vi "PH_ImageOperator.write PSDB Position data.vi"(0 "i ref in":refnum<vi>, 5 "error in":errorcluster) -> (14 "i ref out":refnum<vi>, 16 "Position Boolean data":T1[](array[typedef]), 17 "Position Numeric data":T3[](array[typedef]), 18 "Position String data":T2[](array[typedef]), 19 "error out":errorcluster)   [LabVIEW 2014, in "PH_ImageOperator.lvlib"]
uses:
  PH_ImageOperator.lvlib
  PH_PSDBWriter/PH_PSDBWriter.Numeric dataset.ctl
  PH_PSDBWriter/PH_PSDBWriter.String dataset.ctl
  PH_PSDBWriter/PH_PSDBWriter.Boolean dataset.ctl
  PH_StatusHandler/PH_StatusHandler.Status.ctl
  PH_PSDBWriter/PH_PSDBWriter.lvlib
  PH_StatusHandler/PH_StatusHandler.lvlib
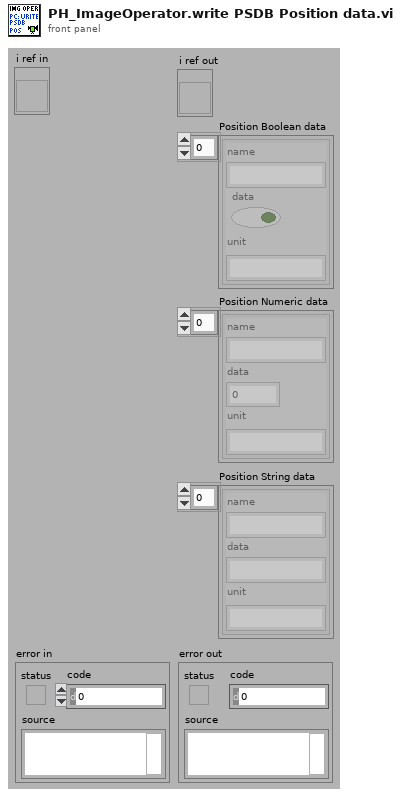
[diagram p1: front panel]
types:
  T1 = typedef "PH_PSDBWriter.lvlib/PH_PSDBWriter.Boolean dataset.ctl" = cluster{"name":string, "data":bool, "unit":string}
  T2 = typedef "PH_PSDBWriter.lvlib/PH_PSDBWriter.String dataset.ctl" = cluster{"name":string, "data":string, "unit":string}
  T3 = typedef "PH_PSDBWriter.lvlib/PH_PSDBWriter.Numeric dataset.ctl" = cluster{"name":string, "data":dbl, "unit":string}
  T4 = typedef "PH_ImageOperator.lvlib/PH_ImageOperator.i attribute.ctl" = cluster{"GUI Refs":cluster{"Delete":refnum<vi>, "Calibration status":refnum<vi>, "BI subtracted":refnum<vi>, "calc Energy":refnum<vi>, "Energy: expected value":refnum<vi>, "Energy: Tolerance":refnum<vi>, "Energy calculated":refnum<vi>, "Energy":refnum<vi>, "calc Beam Anal":refnum<vi>, "Maj Diam 1/esquare":refnum<vi>, "Min Diam 1/esquare":refnum<vi>, "Azi Angle":refnum<vi>, "Min/Maj Diam esquare":refnum<vi>, "Beam analysed":refnum<vi>, "CoG - x":refnum<vi>, "CoG - y":refnum<vi>, "BA: Method":refnum<vi>, "BA: Steps":refnum<vi>, "BA: Factor":refnum<vi>, "calc Traces":refnum<vi>, "Traces: Fit Gauss":refnum<vi>, "Traces calculated":refnum<vi>, "Maj FWHM":refnum<vi>, "Min FWHM":refnum<vi>, "Major Trace":refnum<vi>, "Minor Trace":refnum<vi>, "Maj Fit Order":refnum<vi>, "Min Fit Order":refnum<vi>, "Position calculated":refnum<vi>, "Position":refnum<vi>, "Type":refnum<vi>, "Center":refnum<vi>, "exp - X":refnum<vi>, "exp - Y":refnum<vi>, "Tolerance":refnum<vi>, "f":refnum<vi>, "M":refnum<vi>, "D":refnum<vi>, "q":refnum<vi>, "Dummy Method":refnum<vi>, "Dummy Type":refnum<vi>, "Global On":refnum<vi>, "Traces: No offset":refnum<vi>, "Maj 99%":refnum<vi>, "Min 99%":refnum<vi>, "GUI FF Image":refnum<vi>, "calc Fill Factor":refnum<vi>, "FF calculated":refnum<vi>, "Fill Factor: Filter?":refnum<vi>, "FF: Damage Threshold":refnum<vi>, "FF: Threshold":refnum<vi>, "FF: max allow. Energy":refnum<vi>, "FF: Fillfactor":refnum<vi>, "Calibration data":refnum<vi>}, "List of GUIs":string[], "Calibration":cluster{"Status":T5, "Calibration data":T6, "Calibration Data File":path}, "Final Image":cluster{"BI Subtraction Failure":bool}, "Energy":cluster{"on":bool, "expected value [mJ]":dbl, "Tolerance [%]":dbl, "State":T5, "Energy [mJ]":dbl, "Unit":string, "calculated @":timestamp}, "Beam Analysis":cluster{"on":bool, "Data":T7, "Method":bool, "Steps":i32, "Factor":i32, "ROI":cluster{"Left":i32, "Top":i32, "Right":i32, "Bottom":i32}, "analysed @":timestamp}, "Trace Analysis":cluster{"on":bool, "Fit on":bool, "Maj FWHM":dbl, "Min FWHM":dbl, "Maj Fit Order":i32, "Min Fit Order":i32, "No Offset":bool, "Maj 99%":dbl, "Min 99%":dbl, "Traces":cluster{"XScaleName":string, "Y Scale Minimum":sgl, "Y Scale Maximum":sgl, "X Scale Minimum":sgl, "X Scale Maximum":sgl, "Traces":cluster{"Index":sgl[], "Trace":dbl[]}[]}[], "analysed @":timestamp}, "Position Analysis":cluster{"on":bool, "exp - X":i32, "exp - Y":i32, "focal length [mm]":dbl, "Magnification":dbl, "Delta":dbl, "Theta":dbl, "Tolerance":dbl, "Type":bool, "analysed @":timestamp}, "Fill Factor":cluster{"on":bool, "Filter on?":bool, "Threshold":dbl, "Damage Threshold [J/cm²]":dbl, "Fillfactor":dbl, "Max. allowed Energy [J]":dbl, "calculated @":timestamp}, "Statistician Service ID":i32, "Images":cluster{"Background":T8, "OP":T8, "GUI":T8, "BA: ROI":T8, "Trace: Turn":T8, "FF: Main":T8, "FF: Help":T8, "PSDB: BG":T8, "PSDB: OP":T8, "PSDB: FF":T8}}
  T5 = typedef "PH_StatusHandler.lvlib/PH_StatusHandler.Status.ctl" = i16
  T6 = typedef "PH_ImageCalibrator.lvlib/PH_ImageCalibrator.Calibration Data.ctl" = cluster{"Date":string, "Time":string, "Cam Settings":cluster{"Cam ID":string, "Gain":dbl, "Brightness":dbl, "Shutter":dbl, "Cam Error":bool, "Mode":i32}, "Background Image":cluster{"Image":dbl[][], "Image Error":bool}, "Linear Calibration":cluster{"Calibration Factor":dbl, "not mm or mrad":bool}, "Energy Calibration":cluster{"Calibration Factor":dbl, "no mJ":bool}}
  T7 = typedef "PH_ImageOperator.lvlib/PH_ImageOperator.Beam Analysis Data.ctl" = cluster{"CoG-x":sgl, "CoG-y":sgl, "Maj Dim":dbl, "Min Dim":dbl, "Ellipticity":dbl, "Azimuth Angle [rad]":dbl, "Azi Angle rel to Maj?":bool}
  T8 = typedef "IMAQ Image.ctl" = refnum<image>
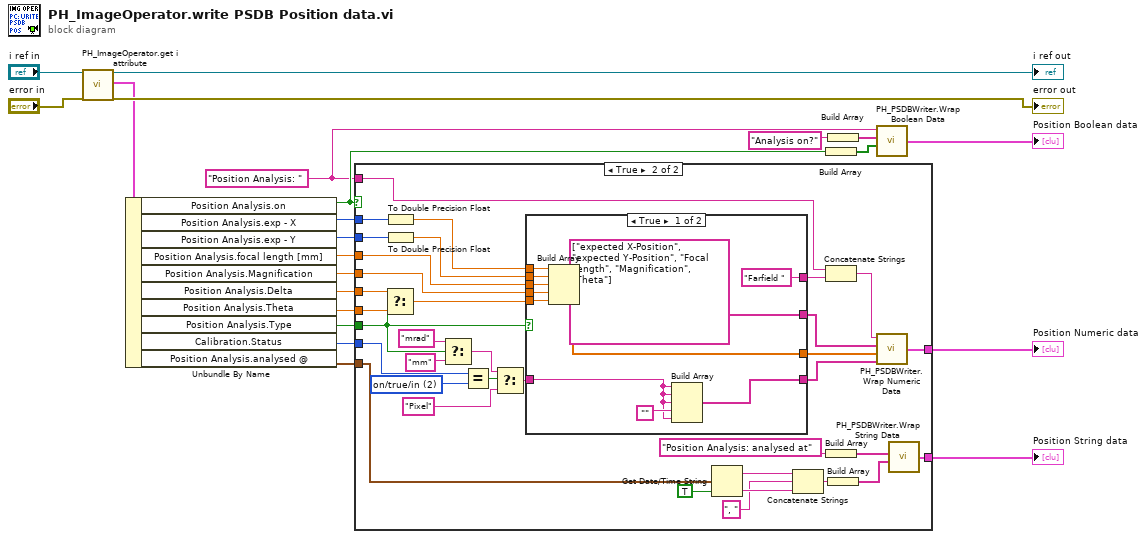
[diagram p0: block diagram]
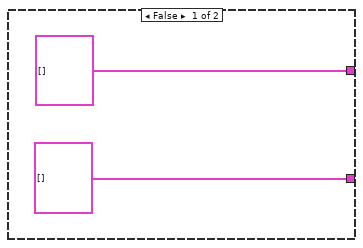
[diagram p2: hidden frame]
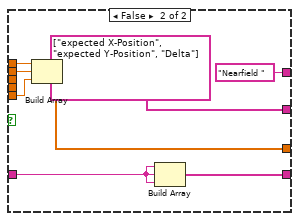
[diagram p3: hidden frame]
diagram:
  w3 = "Position Analysis: " ("string")
  n1 = call "PH_ImageOperator.get i attribute.vi"("i ref in"="i ref in", "error in (no error)"="error in") -> ("i ref out"=→"i ref out":refnum<vi>, "i attribute"=w17:T4, "error out"=→"error out":errorcluster)  [unwired: 15 in]
  n2 = Unbundle By Name(w17) -> ("Position Analysis.on"=w6:bool, "Position Analysis.exp - X"=w16:i32, "Position Analysis.exp - Y"=w15:i32, "Position Analysis.focal length [mm]"=w14:dbl, "Position Analysis.Magnification"=w13:dbl, "Position Analysis.Delta"=w12:dbl, "Position Analysis.Theta"=w11:dbl, "Position Analysis.Type"=w10:bool, "Calibration.Status"=w9:T5, "Position Analysis.analysed @"=w8:timestamp)
  n3 = case shown="True" w6 {
    tunnel: w16 -> [_ w48]
    tunnel: w15 -> [_ w50]
    tunnel: w14 -> [_ w51]
    tunnel: w13 -> [_ w52]
    tunnel: w12 -> [_ w45]
    tunnel: w11 -> [_ w46]
    tunnel: w10 -> [_ w43]
    tunnel: [T3[] [] w25] -> w18
    tunnel: w9 -> [_ w56]
    tunnel: w8 -> [_ w36]
    tunnel: [T2[] [] w34] -> w7
    tunnel: w3 -> [_ w35]
    frame False {
    }
    frame True {
      w59 = T5 2 items=["no info", "off/false/out", "on/true/in", "Failure", "Alarm", "Status 1", "Status 2", "Status 3"] ("Calibration.Status")
      n4 = Select(t=w45, s=w43, f=w46) -> (s? t:f=w44:dbl)
      n5 = To Double Precision Float(number=w48) -> (double precision float=w47:dbl)
      n6 = To Double Precision Float(number=w50) -> (double precision float=w49:dbl)
      n7 = Select(t="mrad" ("string"), s=w43, f="mm") -> (s? t:f=w53:string)
      n8 = Equal?(x=w56, y=w59) -> (x = y?=w58:bool)
      n9 = Select(t=w53, s=w58, f="Pixel" ("string")) -> (s? t:f=w41:string)
      n10 = case shown="True" w43 {
        tunnel: [string[] ["expected X-Position", "expected Y-Position", "Focal Length", "Magnification", "Theta"] string[] ["expected X-Position", "expected Y-Position", "Delta"]] -> w27
        tunnel: [w69 w77] -> w28
        tunnel: w52 -> [w68 _]
        tunnel: w51 -> [w67 _]
        tunnel: w49 -> [w66 w76]
        tunnel: w47 -> [w65 w75]
        tunnel: w44 -> [w64 w71]
        tunnel: ["Farfield " ("string") "Nearfield " ("string")] -> w42
        tunnel: w41 -> [w61 w73]
        tunnel: [w60 w72] -> w29
        frame True {
          n11 = Build Array(w65, w66, w67, w68, w64) -> (w69:dbl[])
          n12 = Build Array(w61, w61, w61, "", w61) -> (w60:string[])
        }
        frame False {
          n13 = Build Array(w75, w76, w71) -> (w77:dbl[])
          n14 = Build Array(w73, w73, w73) -> (w72:string[])
        }
      }
      n15 = Get Date/Time String(seconds (now)=w36, want seconds? (F)=TRUE) -> (date string=w38:string, time string=w40:string)  [unwired: 1 in]
      n16 = Concatenate Strings(w38, ", " ("string"), w40) -> (w32:string)
      n17 = Concatenate Strings(w35, w42) -> (w26:string)
      n18 = Build Array("Position Analysis: analysed at" ("string")) -> (w31:string[])
      n19 = Build Array(w32) -> (w30:string[])
      n20 = call "PH_PSDBWriter.Wrap Numeric Data.vi"("Unit Array"=w29, "Data Array"=w28, "Name Array"=w27, "Name Prefix"=w26) -> ("PSDB Numeric Data Array"=w25:T3[])
      n21 = call "PH_PSDBWriter.Wrap String Data.vi"("Data Array"=w30, "Name Array"=w31) -> ("PSDB String Data Array"=w34:T2[])  [unwired: 2 in]
    }
  }
  "Position Numeric data" <- w18
  "Position String data" <- w7
  n22 = Build Array(w6) -> (w4:bool[])
  n23 = Build Array("Analysis on?" ("name")) -> (w1:string[])
  n24 = call "PH_PSDBWriter.Wrap Boolean Data.vi"("Data Array"=w4, "Name Array"=w1, "Name Prefix"=w3) -> ("PSDB Boolean Data Array"=→"Position Boolean data":T1[])  [unwired: 1 in]
